vi "Get list of Experiment Lines.vi"(8 "error in (no error)":errorcluster, 10 "This vi ref":refnum<vi>, 11 "menu reference":refnum<k9>) -> (0 "error out":errorcluster, 3 "Experiment Lines":string[](array[string]))   [LabVIEW 2020]
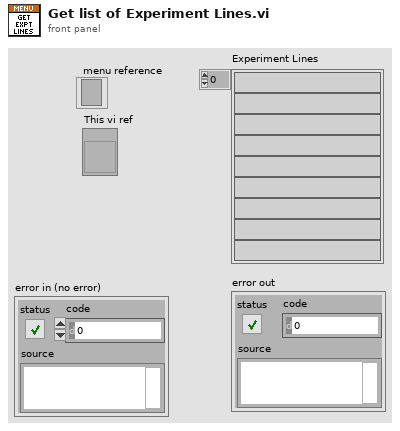
[diagram p1: front panel]
types:
  T1 = typedef "mysql_authentication.ctl" = cluster{"User":string, "Password":string, "Database":string}
  T2 = cluster{"Port":u16, "IP Address":string, "Authentication":T1}
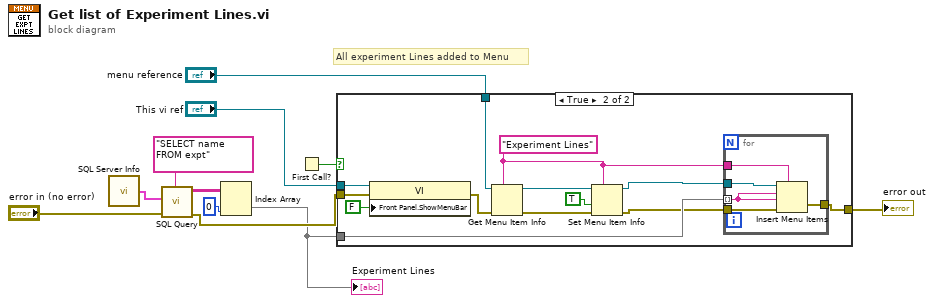
[diagram p0: block diagram]
diagram:
  # "All experiment Lines added to Menu"
  n1 = call "SQL Server Info.vi"() -> ("SQL Server Info"=w9:T2)
  n2 = call "SQL Query.vi"("error in (no error)"="error in (no error)", "SQL Server Info"=w9, "Query"="SELECT name FROM expt") -> ("error out"=w4:errorcluster, "data"=w10:string[][])  [unwired: 7 in]
  n3 = Index Array(array=w10, index (col)=0 ("disabled index (col)")) -> (element=w1:string[])  [unwired: 1 in]
  "Experiment Lines" <- w1
  n4 = First Call?() -> (First Call?: T/F=w2:bool)
  n5 = case shown="True" w2 {
    tunnel: w1 -> [_ w25]
    tunnel: [w12 w19] -> w7
    tunnel: "menu reference" -> [_ w18]
    tunnel: w4 -> [w12 w15]
    tunnel: "This vi ref" -> [_ w13]
    frame False {
    }
    frame True {
      w17 = "Experiment Lines" ("item tag")
      n6 = property class="VI"(reference=w13, error in=w15, "Front Panel.ShowMenuBar"=FALSE ("Front Panel Window:Show Menu Bar")) -> (error out=w14:errorcluster)  [unwired: 1 out]
      n7 = Get Menu Item Info(7:w17, 8:w14, 11:w18) -> (0:w24:errorcluster, 3:w20:refnum<k9>)  [unwired: 5 out]
      n8 = Set Menu Item Info(7:w17, 8:w24, 9:TRUE ("enabled"), 11:w20) -> (0:w23:errorcluster, 3:w22:refnum<k9>)  [unwired: 3 in]
      n9 = for {
        tunnel: w25 -> [w30] mode=indexing
        tunnel: w22 -> [w29]
        tunnel: [w28] -> w19
        tunnel: w23 -> [w27]
        tunnel: w17 -> [w26]
        n10 = Insert Menu Items(5:w26, 6:w27, 7:w30, 8:w30, 9:w29) -> (0:w28:errorcluster)  [unwired: 1 in, 2 out]
      }
    }
  }
  "error out" <- w7
